vi "OpenBoard.vi"(8 "error in (no error)":errorcluster, 10 "Board Address":i8 max=31, 11 "VISA resource name":refnum<visa-resource-name>) -> (0 "error out":errorcluster, 3 "BoardHandle":T1)   [LabVIEW 2020, in "CAEN PSM.lvlib"]
doc: "This function allows to open the device. Therefore, call this VI after calling Initialize.vi.\nYou can need to call this function more times if you use several boards in daisy chain."
uses:
  CAEN PSM.lvlib
  BoardHandle.ctl
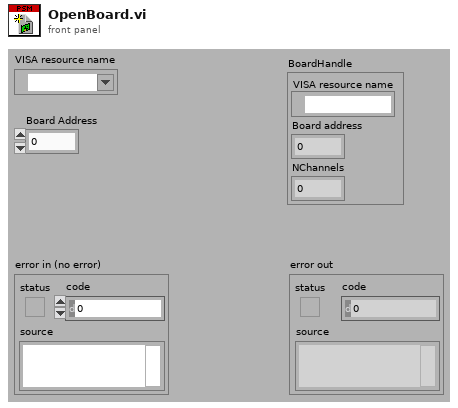
[diagram p1: front panel]
types:
  T1 = typedef "CAEN PSM.lvlib/BoardHandle.ctl" = cluster{"VISA resource name":refnum<visa-resource-name>, "Board address":i8, "NChannels":u8}
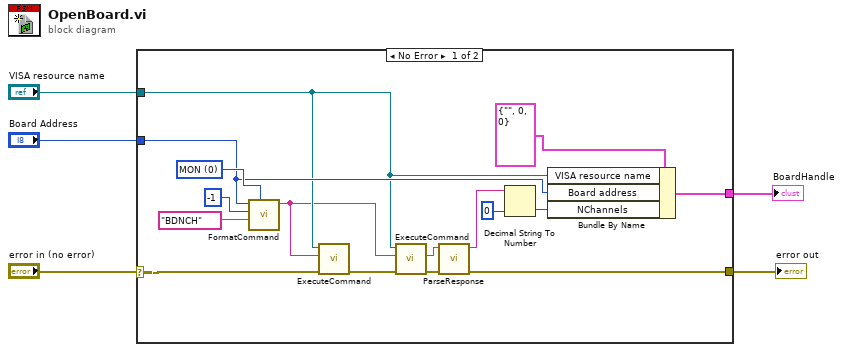
[diagram p0: block diagram]
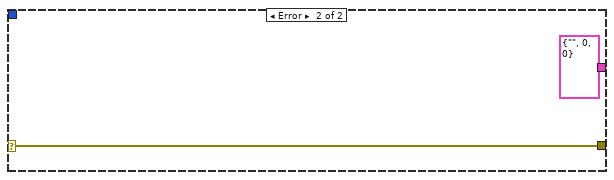
[diagram p2: hidden frame]
diagram:
  n1 = case shown="No Error" "error in (no error)" {
    selector: "error in (no error)" -> [w7 w23]
    tunnel: "Board Address" -> [w17 _]
    tunnel: [w15 T1 {"VISA resource name"="", "Board address"=0, "NChannels"=0} ("BoardHandle")] -> w4
    tunnel: "VISA resource name" -> [w10 _]
    tunnel: [w6 w23] -> w1
    frame No Error {
      w20 = u8 0 items=["MON", "SET"] ("CMD")
      n2 = call "FormatCommand.vi"("CMD (MON)"=w20, "PAR"="BDNCH", "CH"=i8 -1, "BD (0)"=w17) -> ("cmd"=w8:string)  [unwired: 7 in]
      n3 = call "ExecuteCommand.vi"("error in (no error)"=w7, "Command"=w8, "VISA resource name"=w10) -> ("error out"=w11:errorcluster)  [unwired: 6 in, 2 out]
      n4 = call "ExecuteCommand.vi"("error in (no error)"=w11, "Command"=w8, "VISA resource name"=w10) -> ("error out"=w13:errorcluster, "Response"=w14:string)  [unwired: 6 in, 1 out]
      n5 = call "ParseResponse.vi"("error in (no error)"=w13, "Response"=w14) -> ("error out"=w6:errorcluster, "val"=w12:string)  [unwired: 6 in, 2 out]
      n6 = Decimal String To Number(string=w12, default (0L)=u8 0 ("default (0 I32)")) -> (number=w18:u8)  [unwired: 1 in, 1 out]
      n7 = Bundle By Name(cluster=T1 {"VISA resource name"="", "Board address"=0, "NChannels"=0} ("BoardHandle"), "VISA resource name"=w10, "Board address"=w17, "NChannels"=w18) -> (w15:T1)
    }
    frame Error {
    }
  }
  "BoardHandle" <- w4
  "error out" <- w1
